vi "Read Sensors.vi"(0 "NavX Loop Time (ms)":u32, 2 "General Loop Time (ms)":u32) -> ()   [LabVIEW 2017]
uses:
  Globals/Robot Global Data.vi
  <vilib>/Rock Robotics/Network Tables/NT Write Boolean.vi
  Public/Documents/Cross The Road Electronics/Phoenix-LabVIEW/Motor Controller/Get/CTRE_Phoenix_MotorController_GetPulseWidthAll.vi
  <vilib>/Rock Robotics/Network Tables/NT Write Number.vi
  <vilib>/Rock Robotics/Network Tables/NT Read Boolean.vi
  <vilib>/Rock Robotics/Network Tables/NT Read Number.vi
panel:
  in  "Boolean":bool
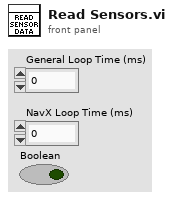
[diagram p1: front panel]
types:
  T1 = cluster{"Rollover":dbl, "Yaw":dbl, "Cont Yaw":dbl}
  T2 = cluster{"Yaw":dbl, "Roll":dbl, "Pitch":dbl, "Heading":dbl, "Fused Heading":dbl}
  T3 = typedef "WPI_SwitchDevRef.ctl" = cluster{"DevStatus":errorcluster, "DIO Channel":T4, "CntIndex":T5, "Normally Closed":bool}
  T4 = typedef "FPGA_DIOChannel.ctl" = enum8{"DIO 0", "DIO 1", "DIO 2", "DIO 3", "DIO 4", "DIO 5", "DIO 6", "DIO 7", "DIO 8", "DIO 9", "DIO MXP 0", "DIO MXP 1", "DIO MXP 2", "DIO MXP 3", "DIO MXP 4", "DIO MXP 5", "DIO MXP 6", "DIO MXP 7", "DIO MXP 8", "DIO MXP 9", "DIO MXP 10", "DIO MXP 11", "DIO MXP 12", "DIO MXP 13", "DIO MXP 14", "DIO MXP 15", "SPI Port CS1", "SPI Port CS2", "SPI Port CS3", "SPI Port MISO", "SPI Port MOSI", "Invalid"}
  T5 = typedef "FPGA_CounterCtrSystemIndex.ctl" = enum8{"Ctr 0", "Ctr 1", "Ctr 2", "Ctr 3", "Ctr 4", "Ctr 5", "Ctr 6", "Ctr 7", "Invalid"}
  T6 = typedef "WPI_EncoderDevRef.ctl" = cluster{"DevStatus":errorcluster, "EncoderIndex":T7, "CounterIndex":T5, "DistancePerCount":dbl, "Decoding Type":T8}
  T7 = typedef "FPGA_EncoderIdx.ctl" = enum8{"Enc 0", "Enc 1", "Enc 2", "Enc 3", "Enc 4", "Enc 5", "Enc 6", "Enc 7", "Invalid"}
  T8 = typedef "WPI_EncoderType.ctl" = enum16{"1x", "2x", "4x"}
  T9 = typedef "WPI_MotorControlDeviceRef.ctl" = cluster{"DeviceStatus":errorcluster, "Type":T10, "PWM":cluster{"PWM Channel":T11, "DeadBand":T12}, "CAN":cluster{"Device Number":u8, "SetOutput VI Ref":variant, "GetOutput VI Ref":variant, "Enable VI Ref":variant, "Disable VI Ref":variant, "Data":variant}, "Invert":bool, "DIO PWM":cluster{"PWM \"Enable\" Channel":T11, "DIOChannel":T4, "PWM Rate":dbl}}
  T10 = typedef "WPI_MotorControlType.ctl" = enum16{"PWM", "CAN", "DIO PWM"}
  T11 = typedef "FPGA_DIOPWMChannel.ctl" = enum8{"PWM 0", "PWM 1", "PWM 2", "PWM 3", "PWM 4", "PWM 5", "PWM 6", "PWM 7", "PWM 8", "PWM 9", "PWM MXP 0", "PWM MXP 1", "PWM MXP 2", "PWM MXP 3", "PWM MXP 4", "PWM MXP 5", "PWM MXP 6", "PWM MXP 7", "PWM MXP 8", "PWM MXP 9", "Invalid"}
  T12 = typedef "WPI_PWMDeadband.ctl" = cluster{"Name":string, "maxPositivePwm":i32, "minPositivePwm":i32, "centerPwm":i32, "maxNegativePwm":i32, "minNegativePwm":i32, "angularRange":u16}
  T13 = typedef "WPI_AnalogChannelDevRef.ctl" = cluster{"DevStatus":errorcluster, "Analog Channel":T14}
  T14 = typedef "FPGA_AIChannel.ctl" = enum8{"AI 0", "AI 1", "AI 2", "AI 3", "AI MXP 0", "AI MXP 1", "AI MXP 2", "AI MXP 3", "Invalid"}
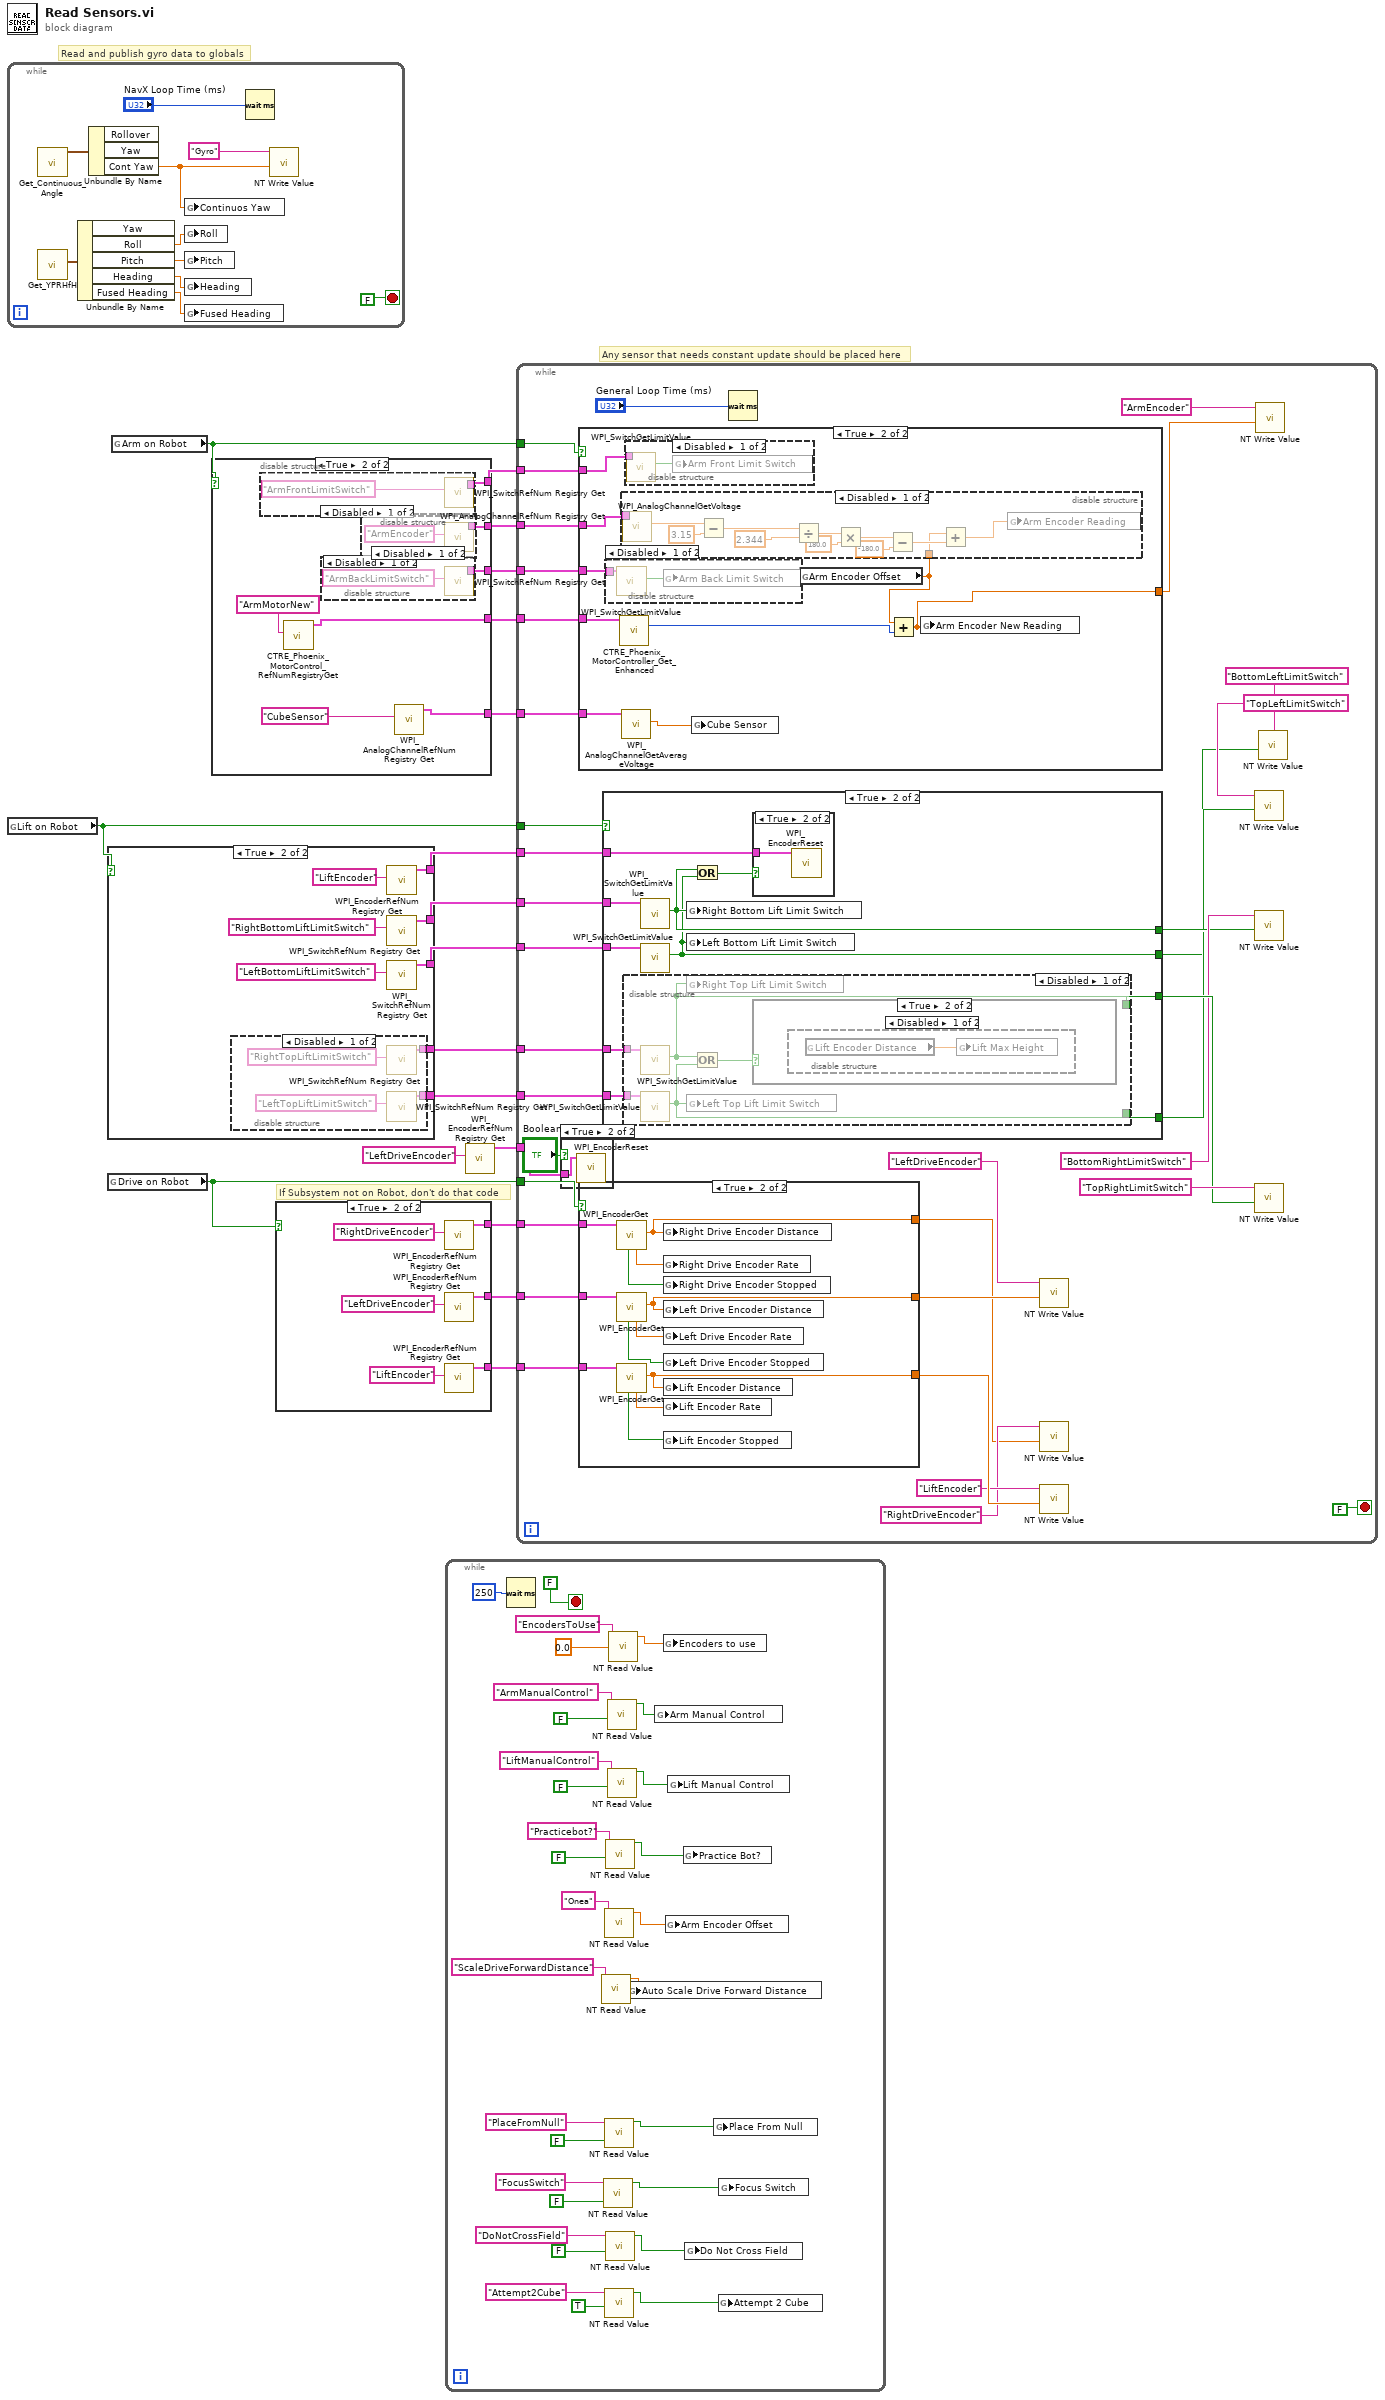
[diagram p0: block diagram]
diagram:
  # "Read and publish gyro data to globals"
  # "If Subsystem not on Robot, don't do that code"
  # "Any sensor that needs constant update should be placed here"
  n1 = while {
    stop <- FALSE stop-if-true
    n2 = call <vilib>:"Get_Continuous_Angle.vi"() -> ("Continuous Angle"=w21:T1)  [unwired: 11 in]
    n3 = call <vilib>:"Get_YPRHfH.vi"() -> ("YRPHfH"=w27:T2)  [unwired: 11 in]
    n4 = Unbundle By Name(w27) -> ("Roll"=w26:dbl, "Pitch"=w25:dbl, "Heading"=w24:dbl, "Fused Heading"=w23:dbl)  [unwired: 1 out]
    n5 = Unbundle By Name(w21) -> ("Cont Yaw"=w20:dbl)  [unwired: 2 out]
    n6 = global write "Robot Global Data.vi" "Continuos Yaw"(w20) -> ()
    n7 = global write "Robot Global Data.vi" "Roll"(w26) -> ()
    n8 = global write "Robot Global Data.vi" "Pitch"(w25) -> ()
    n9 = global write "Robot Global Data.vi" "Heading"(w24) -> ()
    n10 = global write "Robot Global Data.vi" "Fused Heading"(w23) -> ()
    n11 = Wait (ms)(milliseconds to wait="NavX Loop Time (ms)") -> ()  [unwired: 1 out]
    n12 = call-poly <vilib>:"NT Write Value.vi"("Numeric"=w20, "Name"="Gyro") -> ()  [unwired: 9 in, 1 out]
  }
  n13 = global read "Robot Global Data.vi" "Lift on Robot"() -> (w8:bool)
  n14 = case shown="True" w8 {
    tunnel: [_ w36] -> w14
    tunnel: [_ w34] -> w13
    tunnel: [_ w33] -> w12
    tunnel: [_ w32] -> w11
    tunnel: [_ w29] -> w5
    frame False {
    }
    frame True {
      n15 = disable-structure shown="Disabled" {
        disable-tunnel: [w40 _] -> w34
        disable-tunnel: [w39 _] -> w32
        frame Disabled {
          n16 = call <vilib>:"WPI_SwitchRefNum Registry Get.vi"("refnum name"="RightTopLiftLimitSwitch") -> ("SwitchDevRef"=w39:T3)  [unwired: 9 in, 1 out]
          n17 = call <vilib>:"WPI_SwitchRefNum Registry Get.vi"("refnum name"="LeftTopLiftLimitSwitch") -> ("SwitchDevRef"=w40:T3)  [unwired: 9 in, 1 out]
        }
        frame Enabled {
        }
      }
      n18 = call <vilib>:"WPI_EncoderRefNum Registry Get.vi"("refnum name"="LiftEncoder") -> ("EncoderDevRef"=w29:T6)  [unwired: 9 in, 1 out]
      n19 = call <vilib>:"WPI_SwitchRefNum Registry Get.vi"("refnum name"="RightBottomLiftLimitSwitch") -> ("SwitchDevRef"=w33:T3)  [unwired: 9 in, 1 out]
      n20 = call <vilib>:"WPI_SwitchRefNum Registry Get.vi"("refnum name"="LeftBottomLiftLimitSwitch") -> ("SwitchDevRef"=w36:T3)  [unwired: 9 in, 1 out]
    }
  }
  n21 = global read "Robot Global Data.vi" "Drive on Robot"() -> (w6:bool)
  n22 = global read "Robot Global Data.vi" "Arm on Robot"() -> (w7:bool)
  n23 = case shown="True" w7 {
    tunnel: [_ w47] -> w16
    tunnel: [_ w46] -> w10
    tunnel: [_ w45] -> w9
    tunnel: [_ w43] -> w4
    tunnel: [_ w41] -> w3
    frame False {
    }
    frame True {
      n24 = disable-structure shown="Disabled" {
        disable-tunnel: [w51 _] -> w45
        frame Disabled {
          n25 = call <vilib>:"WPI_SwitchRefNum Registry Get.vi"("refnum name"="ArmFrontLimitSwitch") -> ("SwitchDevRef"=w51:T3)  [unwired: 9 in, 1 out]
        }
        frame Enabled {
        }
      }
      n26 = call "CTRE_Phoenix_MotorControl_RefNumRegistryGet.vi"("refnum name"="ArmMotorNew") -> ("PhoenixMotorControlDevRef"=w43:T9)  [unwired: 9 in, 1 out]
      n27 = disable-structure shown="Disabled" {
        disable-tunnel: [w53 _] -> w46
        frame Disabled {
          n28 = call <vilib>:"WPI_SwitchRefNum Registry Get.vi"("refnum name"="ArmBackLimitSwitch") -> ("SwitchDevRef"=w53:T3)  [unwired: 9 in, 1 out]
        }
        frame Enabled {
        }
      }
      n29 = disable-structure shown="Disabled" {
        disable-tunnel: [w49 _] -> w47
        frame Disabled {
          n30 = call <vilib>:"WPI_AnalogChannelRefNum Registry Get.vi"("refnum name"="ArmEncoder") -> ("AIDeviceRef"=w49:T13)  [unwired: 9 in, 1 out]
        }
        frame Enabled {
        }
      }
      n31 = call <vilib>:"WPI_AnalogChannelRefNum Registry Get.vi"("refnum name"="CubeSensor") -> ("AIDeviceRef"=w41:T13)  [unwired: 9 in, 1 out]
    }
  }
  n32 = case shown="True" w6 {
    tunnel: [_ w57] -> w18
    tunnel: [_ w56] -> w17
    tunnel: [_ w54] -> w15
    frame False {
    }
    frame True {
      n33 = call <vilib>:"WPI_EncoderRefNum Registry Get.vi"("refnum name"="RightDriveEncoder") -> ("EncoderDevRef"=w56:T6)  [unwired: 9 in, 1 out]
      n34 = call <vilib>:"WPI_EncoderRefNum Registry Get.vi"("refnum name"="LeftDriveEncoder") -> ("EncoderDevRef"=w57:T6)  [unwired: 9 in, 1 out]
      n35 = call <vilib>:"WPI_EncoderRefNum Registry Get.vi"("refnum name"="LiftEncoder") -> ("EncoderDevRef"=w54:T6)  [unwired: 9 in, 1 out]
    }
  }
  n36 = while {
    stop <- FALSE stop-if-true
    n37 = Wait (ms)(milliseconds to wait=u32 250 ("millisecond timer value")) -> ()  [unwired: 1 out]
    n38 = call-poly <vilib>:"NT Read Value.vi"("Name"="ScaleDriveForwardDistance") -> ("Numeric"=w73:dbl)  [unwired: 9 in, 1 out]
    n39 = call-poly <vilib>:"NT Read Value.vi"("Default Value"=FALSE, "Name"="FocusSwitch") -> ("Boolean"=w65:bool)  [unwired: 8 in, 1 out]
    n40 = call-poly <vilib>:"NT Read Value.vi"("Name"="Onea") -> ("Numeric"=w74:dbl)  [unwired: 9 in, 1 out]
    n41 = call-poly <vilib>:"NT Read Value.vi"("Default Value"=FALSE, "Name"="PlaceFromNull") -> ("Boolean"=w60:bool)  [unwired: 8 in, 1 out]
    n42 = call-poly <vilib>:"NT Read Value.vi"("Default Value"=TRUE, "Name"="Attempt2Cube") -> ("Boolean"=w63:bool)  [unwired: 8 in, 1 out]
    n43 = call-poly <vilib>:"NT Read Value.vi"("Default Value"=FALSE, "Name"="Practicebot?") -> ("Boolean"=w77:bool)  [unwired: 8 in, 1 out]
    n44 = call-poly <vilib>:"NT Read Value.vi"("Default Value"=FALSE, "Name"="DoNotCrossField") -> ("Boolean"=w64:bool)  [unwired: 8 in, 1 out]
    n45 = call-poly <vilib>:"NT Read Value.vi"("Default Value"=FALSE, "Name"="ArmManualControl") -> ("Boolean"=w83:bool)  [unwired: 8 in, 1 out]
    n46 = call-poly <vilib>:"NT Read Value.vi"("Default Value"=FALSE, "Name"="LiftManualControl") -> ("Boolean"=w84:bool)  [unwired: 8 in, 1 out]
    n47 = call-poly <vilib>:"NT Read Value.vi"("Default Value"=0.0, "Name"="EncodersToUse") -> ("Numeric"=w82:dbl)  [unwired: 8 in, 1 out]
    n48 = global write "Robot Global Data.vi" "Auto Scale Drive Forward Distance"(w73) -> ()
    n49 = global write "Robot Global Data.vi" "Arm Manual Control"(w83) -> ()
    n50 = global write "Robot Global Data.vi" "Encoders to use"(w82) -> ()
    n51 = global write "Robot Global Data.vi" "Arm Encoder Offset"(w74) -> ()
    n52 = global write "Robot Global Data.vi" "Lift Manual Control"(w84) -> ()
    n53 = global write "Robot Global Data.vi" "Practice Bot?"(w77) -> ()
    n54 = global write "Robot Global Data.vi" "Do Not Cross Field"(w64) -> ()
    n55 = global write "Robot Global Data.vi" "Place From Null"(w60) -> ()
    n56 = global write "Robot Global Data.vi" "Attempt 2 Cube"(w63) -> ()
    n57 = global write "Robot Global Data.vi" "Focus Switch"(w65) -> ()
  }
  n58 = call <vilib>:"WPI_EncoderRefNum Registry Get.vi"("refnum name"="LeftDriveEncoder") -> ("EncoderDevRef"=w1:T6)  [unwired: 9 in, 1 out]
  n59 = while {
    tunnel: w18 -> [w125]
    tunnel: w17 -> [w124]
    tunnel: w16 -> [w122]
    tunnel: w15 -> [w120]
    tunnel: w14 -> [w119]
    tunnel: w13 -> [w118]
    tunnel: w12 -> [w117]
    tunnel: w11 -> [w116]
    tunnel: w10 -> [w115]
    tunnel: w9 -> [w114]
    tunnel: w8 -> [w113]
    tunnel: w7 -> [w112]
    tunnel: w6 -> [w111]
    tunnel: w5 -> [w110]
    tunnel: w4 -> [w94]
    tunnel: w3 -> [w93]
    tunnel: w1 -> [w90]
    stop <- FALSE stop-if-true
    n60 = case shown="True" "Boolean" {
      tunnel: w90 -> [_ w126]
      frame False {
      }
      frame True {
        n61 = call <vilib>:"WPI_EncoderReset.vi"("EncoderDevRef"=w126) -> ()  [unwired: 9 in, 2 out]
      }
    }
    n62 = case shown="True" w112 {
      tunnel: w122 -> [_ w147]
      tunnel: w115 -> [_ w146]
      tunnel: w114 -> [_ w145]
      tunnel: w94 -> [_ w144]
      tunnel: w93 -> [_ w143]
      tunnel: [_ w140] -> w92
      frame False {
      }
      frame True {
        n63 = disable-structure shown="Disabled" {
          disable-tunnel: w146 -> [w163 _]
          frame Disabled {
            n64 = call <vilib>:"WPI_SwitchGetLimitValue.vi"("SwitchDevRef"=w163) -> ("Switch Pressed"=w162:bool)  [unwired: 8 in, 2 out]
            n65 = global write "Robot Global Data.vi" "Arm Back Limit Switch"(w162) -> ()
          }
          frame Enabled {
          }
        }
        n66 = call-poly "CTRE_Phoenix_MotorController_Get_Enhanced.vi"("PhoenixMotorControlDevRef"=w144) -> ("Pulse Width Position"=w141:i32)  [unwired: 9 in, 5 out]
        n67 = call <vilib>:"WPI_AnalogChannelGetAverageVoltage.vi"("AIDeviceRef"=w143) -> ("Voltage"=w142:dbl)  [unwired: 8 in, 2 out]
        n68 = disable-structure shown="Disabled" {
          disable-tunnel: w145 -> [w161 _]
          frame Disabled {
            n69 = call <vilib>:"WPI_SwitchGetLimitValue.vi"("SwitchDevRef"=w161) -> ("Switch Pressed"=w160:bool)  [unwired: 8 in, 2 out]
            n70 = global write "Robot Global Data.vi" "Arm Front Limit Switch"(w160) -> ()
          }
          frame Enabled {
          }
        }
        n71 = global write "Robot Global Data.vi" "Cube Sensor"(w142) -> ()
        n72 = global read "Robot Global Data.vi" "Arm Encoder Offset"() -> (w139:dbl)
        n73 = disable-structure shown="Disabled" {
          disable-tunnel: w147 -> [w159 _]
          disable-tunnel: w139 -> [w148 _]
          frame Disabled {
            n74 = call <vilib>:"WPI_AnalogChannelGetVoltage.vi"("AIDeviceRef"=w159) -> ("Voltage"=w158:dbl)  [unwired: 8 in, 2 out]
            n75 = Subtract(x=w158, y=3.15) -> (x-y=w152:dbl)
            n76 = Divide(x=w152, y=2.344) -> (x/y=w155:dbl)
            n77 = Multiply(x=w155, y=180.0) -> (x*y=w149:dbl)
            n78 = Subtract(x=w149, y=-180.0) -> (x-y=w151:dbl)
            n79 = Add(x=w148, y=w151) -> (x+y=w150:dbl)
            n80 = global write "Robot Global Data.vi" "Arm Encoder Reading"(w150) -> ()
          }
          frame Enabled {
          }
        }
        n81 = Add(x=w139, y=w141) -> (x+y=w140:dbl)
        n82 = global write "Robot Global Data.vi" "Arm Encoder New Reading"(w140) -> ()
      }
    }
    n83 = case shown="True" w111 {
      tunnel: w125 -> [_ w138]
      tunnel: w124 -> [_ w137]
      tunnel: w120 -> [_ w131]
      tunnel: [_ w129] -> w109
      tunnel: [_ w128] -> w105
      tunnel: [_ w127] -> w104
      frame False {
      }
      frame True {
        n84 = call <vilib>:"WPI_EncoderGet.vi"("EncoderDevRef"=w137) -> ("Distance"=w127:dbl, "Rate"=w134:dbl, "Stopped"=w133:bool)  [unwired: 5 in, 3 out]
        n85 = call <vilib>:"WPI_EncoderGet.vi"("EncoderDevRef"=w138) -> ("Distance"=w128:dbl, "Rate"=w136:dbl, "Stopped"=w135:bool)  [unwired: 5 in, 3 out]
        n86 = call <vilib>:"WPI_EncoderGet.vi"("EncoderDevRef"=w131) -> ("Distance"=w129:dbl, "Rate"=w132:dbl, "Stopped"=w130:bool)  [unwired: 5 in, 3 out]
        n87 = global write "Robot Global Data.vi" "Right Drive Encoder Distance"(w127) -> ()
        n88 = global write "Robot Global Data.vi" "Right Drive Encoder Rate"(w134) -> ()
        n89 = global write "Robot Global Data.vi" "Right Drive Encoder Stopped"(w133) -> ()
        n90 = global write "Robot Global Data.vi" "Left Drive Encoder Distance"(w128) -> ()
        n91 = global write "Robot Global Data.vi" "Left Drive Encoder Rate"(w136) -> ()
        n92 = global write "Robot Global Data.vi" "Left Drive Encoder Stopped"(w135) -> ()
        n93 = global write "Robot Global Data.vi" "Lift Encoder Distance"(w129) -> ()
        n94 = global write "Robot Global Data.vi" "Lift Encoder Rate"(w132) -> ()
        n95 = global write "Robot Global Data.vi" "Lift Encoder Stopped"(w130) -> ()
      }
    }
    n96 = case shown="True" w113 {
      tunnel: w119 -> [_ w173]
      tunnel: w118 -> [_ w172]
      tunnel: w117 -> [_ w171]
      tunnel: w116 -> [_ w170]
      tunnel: w110 -> [_ w168]
      tunnel: [_ w167] -> w102
      tunnel: [_ w166] -> w98
      tunnel: [_ w165] -> w97
      tunnel: [_ w164] -> w96
      frame False {
      }
      frame True {
        n97 = disable-structure shown="Disabled" {
          disable-tunnel: w172 -> [w178 _]
          disable-tunnel: w170 -> [w177 _]
          disable-tunnel: [w175 _] -> w167
          disable-tunnel: [w174 _] -> w165
          frame Disabled {
            n98 = call <vilib>:"WPI_SwitchGetLimitValue.vi"("SwitchDevRef"=w177) -> ("Switch Pressed"=w175:bool)  [unwired: 8 in, 2 out]
            n99 = call <vilib>:"WPI_SwitchGetLimitValue.vi"("SwitchDevRef"=w178) -> ("Switch Pressed"=w174:bool)  [unwired: 8 in, 2 out]
            n100 = global write "Robot Global Data.vi" "Right Top Lift Limit Switch"(w175) -> ()
            n101 = global write "Robot Global Data.vi" "Left Top Lift Limit Switch"(w174) -> ()
            n102 = Or(x=w175, y=w174) -> (x .or. y?=w176:bool)
            n103 = case shown="True" w176 {
              frame False {
              }
              frame True {
                n104 = disable-structure shown="Disabled" {
                  frame Disabled {
                    n105 = global read "Robot Global Data.vi" "Lift Encoder Distance"() -> (w179:dbl)
                    n106 = global write "Robot Global Data.vi" "Lift Max Height"(w179) -> ()
                  }
                  frame Enabled {
                  }
                }
              }
            }
          }
          frame Enabled {
          }
        }
        n107 = call <vilib>:"WPI_SwitchGetLimitValue.vi"("SwitchDevRef"=w171) -> ("Switch Pressed"=w166:bool)  [unwired: 8 in, 2 out]
        n108 = call <vilib>:"WPI_SwitchGetLimitValue.vi"("SwitchDevRef"=w173) -> ("Switch Pressed"=w164:bool)  [unwired: 8 in, 2 out]
        n109 = global write "Robot Global Data.vi" "Right Bottom Lift Limit Switch"(w166) -> ()
        n110 = global write "Robot Global Data.vi" "Left Bottom Lift Limit Switch"(w164) -> ()
        n111 = Or(x=w166, y=w164) -> (x .or. y?=w169:bool)
        n112 = case shown="True" w169 {
          tunnel: w168 -> [_ w180]
          frame False {
          }
          frame True {
            n113 = call <vilib>:"WPI_EncoderReset.vi"("EncoderDevRef"=w180) -> ()  [unwired: 9 in, 2 out]
          }
        }
      }
    }
    n114 = Wait (ms)(milliseconds to wait="General Loop Time (ms)") -> ()  [unwired: 1 out]
    n115 = call-poly <vilib>:"NT Write Value.vi"("Numeric"=w105, "Name"="LeftDriveEncoder") -> ()  [unwired: 9 in, 1 out]
    n116 = call-poly <vilib>:"NT Write Value.vi"("Numeric"=w104, "Name"="RightDriveEncoder") -> ()  [unwired: 9 in, 1 out]
    n117 = call-poly <vilib>:"NT Write Value.vi"("Numeric"=w109, "Name"="LiftEncoder") -> ()  [unwired: 9 in, 1 out]
    n118 = call-poly <vilib>:"NT Write Value.vi"("Boolean"=w97, "Name"="TopLeftLimitSwitch") -> ()  [unwired: 9 in, 1 out]
    n119 = call-poly <vilib>:"NT Write Value.vi"("Boolean"=w98, "Name"="BottomRightLimitSwitch") -> ()  [unwired: 9 in, 1 out]
    n120 = call-poly <vilib>:"NT Write Value.vi"("Boolean"=w102, "Name"="TopRightLimitSwitch") -> ()  [unwired: 9 in, 1 out]
    n121 = call-poly <vilib>:"NT Write Value.vi"("Numeric"=w92, "Name"="ArmEncoder") -> ()  [unwired: 9 in, 1 out]
    n122 = call-poly <vilib>:"NT Write Value.vi"("Boolean"=w96, "Name"="BottomLeftLimitSwitch") -> ()  [unwired: 9 in, 1 out]
  }
